vi "Time.vi"() -> ()   [LabVIEW 2012]
panel:
  out "double precision float":dbl
  in  "stop":bool
  out "extended precision float":ext
  in  "End time":timestamp
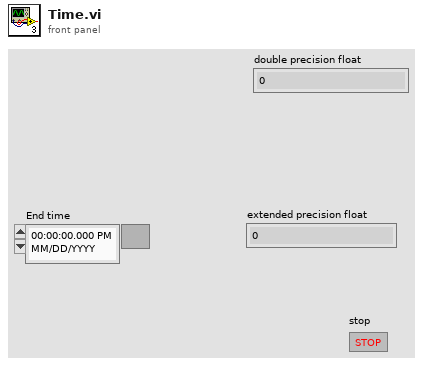
[diagram p1: front panel]
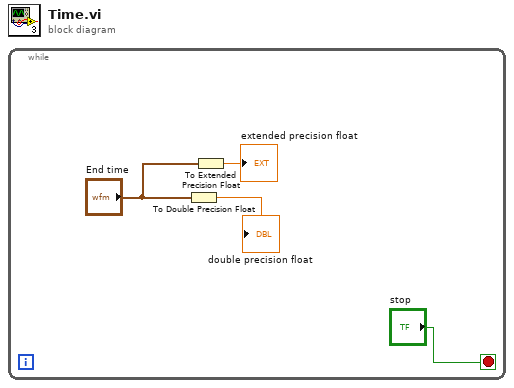
[diagram p0: block diagram]
diagram:
  n1 = while {
    stop <- "stop" stop-if-true
    n2 = To Double Precision Float(number="End time") -> (double precision float=→"double precision float":dbl)
    n3 = To Extended Precision Float(1:"End time") -> (0:→"extended precision float":ext)
  }
